vi "含200行程步进电机查询坐标.vi"(9 "细分设置":dbl=8.0, 10 "查询坐标轴":string, 11 "串口通信端口":refnum<visa-resource-name>) -> (3 "坐标(mm)":dbl)   [LabVIEW 2016]
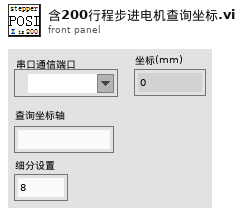
[diagram p1: front panel]
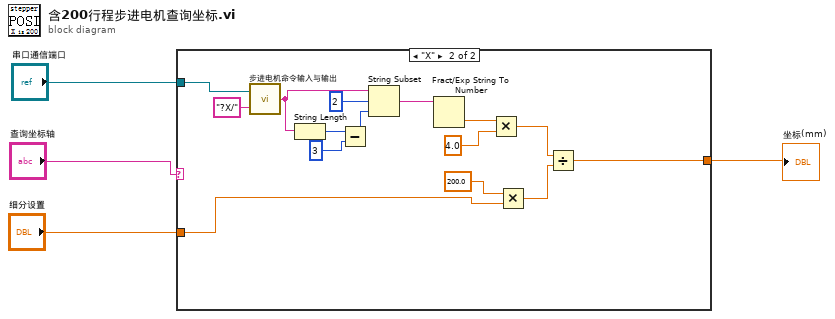
[diagram p0: block diagram]
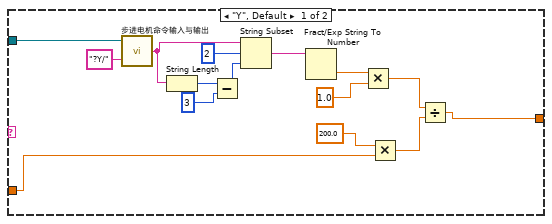
[diagram p2: hidden frame]
diagram:
  n1 = case shown="\"X\"" "查询坐标轴" {
    tunnel: "串口通信端口" -> [w7 w22]
    tunnel: "细分设置" -> [w6 w21]
    tunnel: [w5 w20] -> w1
    frame "Y", Default {
      n2 = call "步进电机命令输入与输出.vi"("输入字符串"="?Y/", "串口通信端口"=w7) -> ("返回字符串"=w12:string)
      n3 = String Length(string=w12) -> (length=w10:i32)
      n4 = Subtract(x=w10, y=3) -> (x-y=w13:i32)
      n5 = String Subset(string=w12, offset (0)=2 ("偏移量(0)"), length (rest)=w13) -> (substring=w14:string)
      n6 = Fract/Exp String To Number(string=w14) -> (number=w15:dbl)  [unwired: 4 out]
      n7 = Multiply(x=w15, y=1.0) -> (x*y=w19:dbl)
      n8 = Multiply(x=200.0, y=w6) -> (x*y=w18:dbl)
      n9 = Divide(x=w19, y=w18) -> (x/y=w5:dbl)
    }
    frame "X" {
      n10 = call "步进电机命令输入与输出.vi"("输入字符串"="?X/", "串口通信端口"=w22) -> ("返回字符串"=w30:string)
      n11 = String Length(string=w30) -> (length=w32:i32)
      n12 = Subtract(x=w32, y=3) -> (x-y=w29:i32)
      n13 = String Subset(string=w30, offset (0)=2 ("偏移量(0)"), length (rest)=w29) -> (substring=w28:string)
      n14 = Fract/Exp String To Number(string=w28) -> (number=w27:dbl)  [unwired: 4 out]
      n15 = Multiply(x=w27, y=4.0) -> (x*y=w23:dbl)
      n16 = Multiply(x=200.0, y=w21) -> (x*y=w24:dbl)
      n17 = Divide(x=w23, y=w24) -> (x/y=w20:dbl)
    }
  }
  "坐标(mm)" <- w1
